vi "StepperStart.vi"(0 "Device Info":T2={"Serial Number"=-1, "Channel"=0, "Port"=0}, 1 "Engaged":bool=TRUE, 5 "Stepper Initialization Data":T1={"Control Mode"=0, " Rescale Factor"=1.0, "Velocity Limit"=10000.0, "Acceleration"=10000.0, "Current Limit"=1.0} {"Control Mode" items=["Step", "Run"]}, 11 "error in (no error)":errorcluster, 12 "Connection":u16(ring) items=["No Preference", "Remote", "Local"], 13 "Timeout (mSec)":i32=5000) -> (4 "Phidget ID":u64, 6 "Serial Number Return":i32, 10 "Attached?":bool, 15 "error out":errorcluster)   [LabVIEW 2020, in "Phidget Stepper.lvlib"]
doc: "${Stepper:StartHeader}"
uses:
  <instrlib>/Phidgets/Phidget Stepper/Phidget Stepper.lvlib
  <instrlib>/Phidgets/Phidget Common/Phidget Common.lvlib
panel:
  # "NOTE: The default Velocity Limit and\nAcceleration parameters will not\nwork with the 1062. These may be\nboth set to 200 (or any other value \nin the valid range) for the device to\nwork."
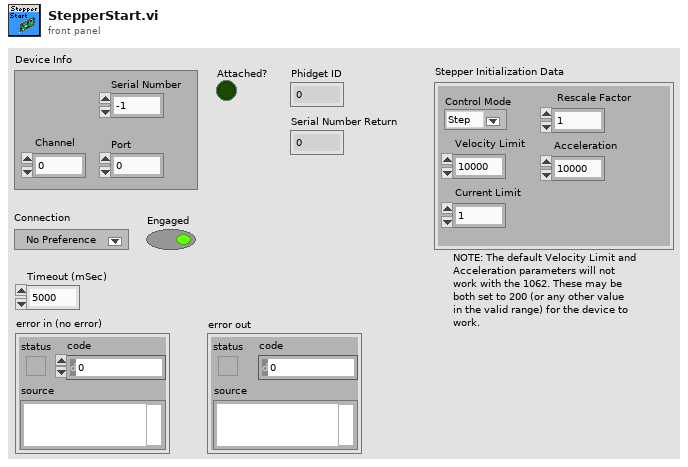
[diagram p1: front panel]
types:
  T1 = cluster{"Control Mode":u16, " Rescale Factor":dbl, "Velocity Limit":dbl, "Acceleration":dbl, "Current Limit":dbl}
  T2 = cluster{"Serial Number":i32, "Channel":i32, "Port":i32}
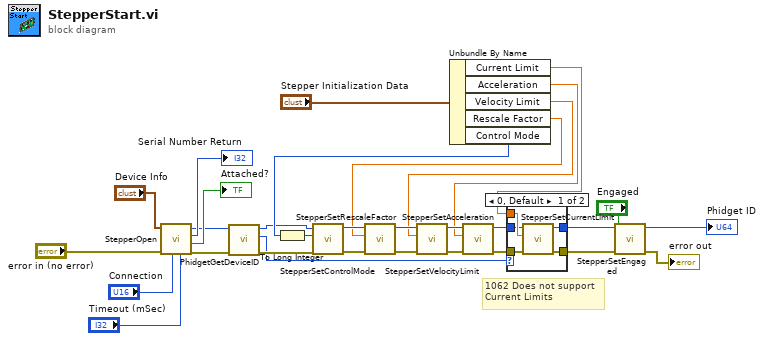
[diagram p0: block diagram]
diagram:
  # "1062 Does not support\nCurrent Limits"
  n1 = call <instrlib>:"StepperOpen.vi"("Timeout (mSec)"="Timeout (mSec)", "Connection"="Connection", "error in"="error in (no error)", "Device Info"="Device Info") -> ("error out"=w6:errorcluster, "Attached?"=→"Attached?":bool, "Serial Number Return"=→"Serial Number Return":i32, "Phidget ID"=w3:u64)  [unwired: 4 in]
  n2 = call <instrlib>:"PhidgetGetDeviceID.vi"("error in (no error)"=w6, "Device In"=w3) -> ("error out"=w5:errorcluster, "Devie IDs"=w1:u32, "Device Out"=w4:u64)  [unwired: 6 in]
  n3 = Unbundle By Name("Stepper Initialization Data") -> ("Current Limit"=w2:dbl, "Acceleration"=w19:dbl, "Velocity Limit"=w20:dbl, "Rescale Factor"=w25:dbl, "Control Mode"=w15:u16)
  n4 = To Long Integer(number=w15) -> (32bit integer=w16:i32)
  n5 = call <instrlib>:"StepperSetControlMode.vi"("error in (no error)"=w5, "Control Mode"=w16, "Device In"=w4) -> ("error out"=w27:errorcluster, "Device Out"=w26:u64)  [unwired: 6 in]
  n6 = call <instrlib>:"StepperSetRescaleFactor.vi"("error in (no error)"=w27, "Rescale Factor"=w25, "Device In"=w26) -> ("error out"=w24:errorcluster, "Device Out"=w23:u64)  [unwired: 6 in]
  n7 = call <instrlib>:"StepperSetVelocityLimit.vi"("error in (no error)"=w24, "Velocity Limit"=w20, "Device In"=w23) -> ("error out"=w21:errorcluster, "Device Out"=w22:u64)  [unwired: 6 in]
  n8 = call <instrlib>:"StepperSetAcceleration.vi"("error in (no error)"=w21, "Acceleration"=w19, "Device In"=w22) -> ("error out"=w17:errorcluster, "Device Out"=w18:u64)  [unwired: 6 in]
  n9 = case shown="0, Default" w1 {
    tunnel: w2 -> [w36 _]
    tunnel: w18 -> [w35 w38]
    tunnel: w17 -> [w34 w37]
    tunnel: [w33 w37] -> w12
    tunnel: [w32 w38] -> w11
    frame 0, Default {
      n10 = call <instrlib>:"StepperSetCurrentLimit.vi"("error in (no error)"=w34, "Current Limit"=w36, "Device In"=w35) -> ("error out"=w33:errorcluster, "Device Out"=w32:u64)  [unwired: 6 in]
    }
    frame 39 {
    }
  }
  n11 = call <instrlib>:"StepperSetEngaged.vi"("error in (no error)"=w12, "Engaged"="Engaged", "Device In"=w11) -> ("error out"=→"error out":errorcluster, "Device Out"=→"Phidget ID":u64)  [unwired: 6 in]
